vi "VMS View.vi"() -> ()   [LabVIEW 2016, in "M1M3SupportEUI_Views.lvlib"]
uses:
  M1M3SupportEUI_Views.lvlib
  Model/Model.lvclass
  SALLV_vms/DataTypes/M1M3.ctl
  SALLV_vms/DataTypes/logevent_AcquisitionRate.ctl
  SALLV_vms/DataTypes/logevent_AppliedSettingsMatchStart.ctl
  SALLV_vms/DataTypes/logevent_ErrorCode.ctl
  SALLV_vms/DataTypes/logevent_SettingVersions.ctl
  SALLV_vms/DataTypes/logevent_SummaryState.ctl
  M1M3 Support Events/M1M3 Support Events.lvclass/M1M3 Support Events.ctl
  M1M3 Support Events/M1M3 Support Events.lvclass
  SALLV_vms/SALLV_vms.lvlib
panel:
  out "VMS Summary State Value":T1(ring)
  out "Recommended Settings Version":string
  out "Error Code":i32
  out "Applied Settings Match Start":bool
  out "Acquisition Rate":dbl
  out "Acquisition Rate Timestamp":timestamp
  out "Stop":bool
  out "logevent_SummaryState":T2
  out "logevent_SettingVersions":T3
  out "logevent_ErrorCode":T4
  out "logevent_AppliedSettingsMatchStart":T5
  out "logevent_AcquisitionRate":T6
  out "Array":dbl[][](array[numeric])
  in  "Topic":string(combo)
  out "Timestamp":timestamp
  out "M1M3":T7
  in  "Model in":refnum<class "Model.lvclass">
  # "VMS"
  # "Data"
  # "0"
  # "1"
  # "2"
  # "3"
  # "4"
  # "5"
  # "6"
  # "7"
  # "8"
  # "9"
  # "00"
  # "10"
  # "20"
  # "30"
  # "40"
  # "Events"
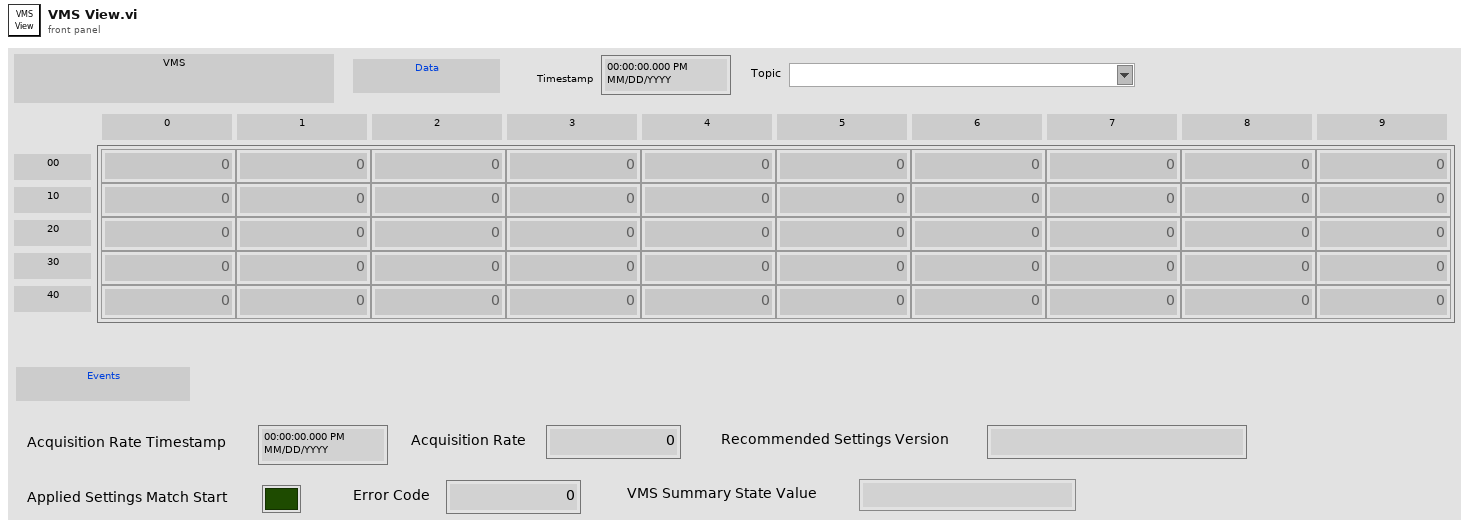
[diagram p1: front panel]
types:
  T1 = enum16{"", "DisabledState", "EnabledState", "FaultState", "OfflineState", "StandbyState"}
  T2 = typedef "SALLV_vms.lvlib/logevent_SummaryState.ctl" = cluster{"SummaryStateValue":enum16{"", "DisabledState", "EnabledState", "FaultState", "OfflineState", "StandbyState"}, "priority":i32}
  T3 = typedef "SALLV_vms.lvlib/logevent_SettingVersions.ctl" = cluster{"recommendedSettingVersion":string, "priority":i32}
  T4 = typedef "SALLV_vms.lvlib/logevent_ErrorCode.ctl" = cluster{"errorCode":i32, "priority":i32}
  T5 = typedef "SALLV_vms.lvlib/logevent_AppliedSettingsMatchStart.ctl" = cluster{"appliedSettingsMatchStartIsTrue":bool, "priority":i32}
  T6 = typedef "SALLV_vms.lvlib/logevent_AcquisitionRate.ctl" = cluster{"Timestamp":dbl, "RateInHz":dbl, "priority":i32}
  T7 = typedef "SALLV_vms.lvlib/M1M3.ctl" = cluster{"Timestamp":dbl, "Sensor1XAcceleration[50]":dbl[], "Sensor1YAcceleration[50]":dbl[], "Sensor1ZAcceleration[50]":dbl[], "Sensor2XAcceleration[50]":dbl[], "Sensor2YAcceleration[50]":dbl[], "Sensor2ZAcceleration[50]":dbl[], "Sensor3XAcceleration[50]":dbl[], "Sensor3YAcceleration[50]":dbl[], "Sensor3ZAcceleration[50]":dbl[]}
  T8 = typedef "M1M3SupportEUI_TypeDefs.lvlib/M1M3 Support Events.ctl" = cluster{"Inclinometer  Data":refnum<user-event>, "IMS Data":refnum<user-event>, "SAL Connected":refnum<user-event>, "Accelerometer Data":refnum<user-event>, "OuterLoop Data":refnum<user-event>, "ErrorCode Event":refnum<user-event>, "InterlockStatus Event":refnum<user-event>, "InterlockWarning Event":refnum<user-event>, "Gyro Data":refnum<user-event>, "HP Actuator Info Event":refnum<user-event>, " FA Info Event":refnum<user-event>, "HP Monitor Info Event":refnum<user-event>, "FA Data":refnum<user-event>, "HP Actuator data":refnum<user-event>, "HP Monitor data":refnum<user-event>, "Air Supply Status Event":refnum<user-event>, "Air Supply Warning Event":refnum<user-event>, "Power Data":refnum<user-event>, "PID Data":refnum<user-event>, "PID Info Event":refnum<user-event>, "Power Status Event":refnum<user-event>, "Power Supply Status Event":refnum<user-event>, "Power Warning Event":refnum<user-event>, "Summary State Event":refnum<user-event>, "Detailed State Event":refnum<user-event>, "FA Force Warning Event":refnum<user-event>, "FA Warning Event":refnum<user-event>, "FA State Event":refnum<user-event>, "Applied AberrationForces Event":refnum<user-event>, "Applied Acceleration Forcces Event":refnum<user-event>, "Applied Azimuth Forces Event":refnum<user-event>, "Applied Active Optic Forces Event":refnum<user-event>, "Applied Balance Forces Event":refnum<user-event>, "Applied Cylinder Forces Event":refnum<user-event>, "Applied Elevation Forces Event":refnum<user-event>, "Applied Forces Event":refnum<user-event>, "Applied Offset Forces Event":refnum<user-event>, "Applied Static Forces Event":refnum<user-event>, "Applied Thermal Forces Event":refnum<user-event>, "Applied Velocity Forces Event":refnum<user-event>, "Rejected Aberration Force Event":refnum<user-event>, "Rejected Acceleration Forces Event":refnum<user-event>, "Rejected Active Optic Forces Event":refnum<user-event>, "Rejected Azimuth Forces Event":refnum<user-event>, "Rejected Balance Forces Event":refnum<user-event>, "Rejected Cylinder Forces Event":refnum<user-event>, "Rejected Elevation Forces Event":refnum<user-event>, "Rejected Forces Event":refnum<user-event>, "Rejected Offset Forces Event":refnum<user-event>, "Rejected Static Forces Event":refnum<user-event>, "Rejected Thermal Forces Event":refnum<user-event>, "Rejected Velocity Forces Event":refnum<user-event>, "Command Rejection Event":refnum<user-event>, "Setting Verions Event":refnum<user-event>, "Settings Applied Event":refnum<user-event>, "HP Actuator State Event":refnum<user-event>, "HP Actuator Warning Event":refnum<user-event>, "HP Monitor State Event":refnum<user-event>, "HP Monitor Warning Event":refnum<user-event>, "Accelerometer Warning Event":refnum<user-event>, "Applied Settings Match Start Event":refnum<user-event>, "Cell Light Status Event ":refnum<user-event>, "Cell Light Warning Event":refnum<user-event>, "Displacement Sensor Warning Event":refnum<user-event>, "Force Setpoint Warning Event":refnum<user-event>, "Gyro Warning Event ":refnum<user-event>, "ILC Warning Event ":refnum<user-event>, "Inclinometer Sensor Warning Event ":refnum<user-event>, "vms M1M3 Data":refnum<user-event>, "vms Acquisition Rate Event":refnum<user-event>, "vms Applied Settings Match Settings Event":refnum<user-event>, "vms Error Code Event":refnum<user-event>, "vms Setting Versions Event":refnum<user-event>, "vms Summary State Event":refnum<user-event>}
  T9 = enum16{"", "DetailedState_DetailedStates_DisabledState", "DetailedState_DetailedStates_EnabledState", "DetailedState_DetailedStates_FaultState", "DetailedState_DetailedStates_OfflineState", "DetailedState_DetailedStates_StandbyState", "DetailedState_DetailedStates_ParkedState", "DetailedState_DetailedStates_RaisingState", "DetailedState_DetailedStates_ActiveState", "DetailedState_DetailedStates_LoweringState", "DetailedState_DetailedStates_EngineeringState", "DetailedState_DetailedStates_ParkedEngineeringState", "DetailedState_DetailedStates_RaisingEngineeringState", "DetailedState_DetailedStates_ActiveEngineeringState", "DetailedState_DetailedStates_LoweringEngineeringState", "DetailedState_DetailedStates_LoweringFaultState", "DetailedState_DetailedStates_ProfileHardpointCorrectionState"}
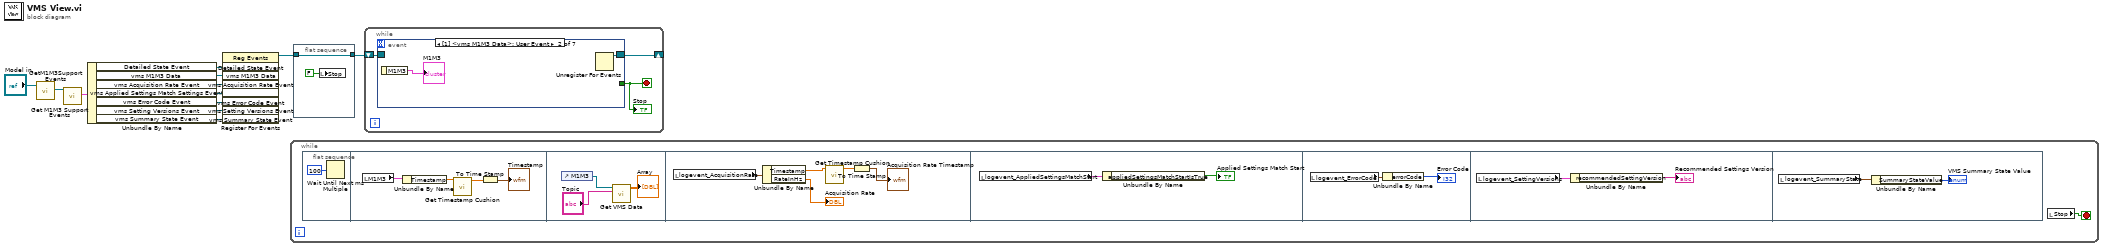
[diagram p0: block diagram]
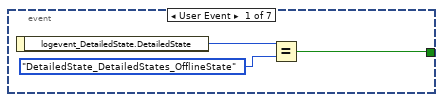
[diagram p2: hidden frame]
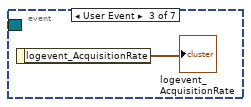
[diagram p3: hidden frame]
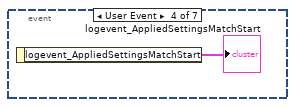
[diagram p4: hidden frame]
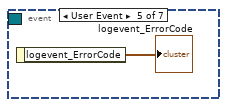
[diagram p5: hidden frame]
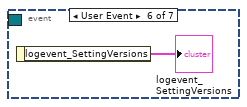
[diagram p6: hidden frame]
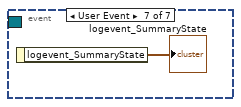
[diagram p7: hidden frame]
diagram:
  n1 = call "GetM1M3SupportEvents.vi"("Model in"="Model in") -> ("M1M3 Support Events out"=w13:refnum<class "M1M3 Support Events.lvclass">)  [unwired: 8 in, 2 out]
  n2 = call "Get M1M3 Support Events.vi"("M1M3 Support Events in"=w13) -> ("M1M3 Support Events"=w11:T8)  [unwired: 9 in, 1 out]
  n3 = Unbundle By Name(w11) -> ("Detailed State Event"=w10:refnum<user-event>, "vms M1M3 Data"=w8:refnum<user-event>, "vms Acquisition Rate Event"=w7:refnum<user-event>, "vms Applied Settings Match Settings Event"=w6:refnum<user-event>, "vms Error Code Event"=w5:refnum<user-event>, "vms Setting Versions Event"=w4:refnum<user-event>, "vms Summary State Event"=w3:refnum<user-event>)
  n4 = register-events(w10, w8, w7, w6, w5, w4, w3) -> (reference out=w2:refnum<event-registration>)  [unwired: 2 in, 1 out]
  n5 = while {
    stop <- w14 stop-if-true
    n6 = flat-sequence {
      frame #0 {
        n7 = Wait Until Next ms Multiple(millisecond multiple=u32 100) -> ()  [unwired: 1 out]
      }
      frame #1 {
        n8 = local read "M1M3"() -> (w19:T7)
        n9 = Unbundle By Name(w19) -> ("Timestamp"=w17:dbl)
        n10 = call "Get Timestamp Cushion.vi"("DoubleTimestampRepresentation"=w17) -> ("TimestampCushion"=w18:dbl)  [unwired: 10 in]
        n11 = To Time Stamp(1:w18) -> (0:→"Timestamp":timestamp)
      }
      frame #2 {
        n12 = control-ref of="M1M3"() -> (w22:refnum<vi>)
        n13 = call "Get VMS Data.vi"("VMS Data Type"="Topic", "Clust Refnum"=w22) -> ("Array"=→"Array":dbl[][])  [unwired: 9 in]
      }
      frame #3 {
        n14 = local read "logevent_AcquisitionRate"() -> (w27:T6)
        n15 = Unbundle By Name(w27) -> ("Timestamp"=w25:dbl, "RateInHz"=→"Acquisition Rate":dbl)
        n16 = call "Get Timestamp Cushion.vi"("DoubleTimestampRepresentation"=w25) -> ("TimestampCushion"=w26:dbl)  [unwired: 10 in]
        n17 = To Time Stamp(1:w26) -> (0:→"Acquisition Rate Timestamp":timestamp)
      }
      frame #4 {
        n18 = local read "logevent_AppliedSettingsMatchStart"() -> (w29:T5)
        n19 = Unbundle By Name(w29) -> ("appliedSettingsMatchStartIsTrue"=→"Applied Settings Match Start":bool)
      }
      frame #5 {
        n20 = local read "logevent_ErrorCode"() -> (w31:T4)
        n21 = Unbundle By Name(w31) -> ("errorCode"=→"Error Code":i32)
      }
      frame #6 {
        n22 = local read "logevent_SettingVersions"() -> (w33:T3)
        n23 = Unbundle By Name(w33) -> ("recommendedSettingVersion"=→"Recommended Settings Version":string)
      }
      frame #7 {
        n24 = local read "logevent_SummaryState"() -> (w35:T2)
        n25 = Unbundle By Name(w35) -> ("SummaryStateValue"=→"VMS Summary State Value":T1)
      }
    }
    n26 = local read "Stop"() -> (w14:bool)
  }
  n27 = flat-sequence {
    tunnel: w2 -> [w37]
    tunnel: [w37] -> w1
    frame #0 {
      n28 = local write "Stop"(FALSE ("Stop")) -> ()
    }
  }
  n29 = while {
    shift-right: [w39] -> w9
    shift-left: w1 -> [w40]
    stop <- w38 stop-if-true
    n30 = event shown="[1] <vms M1M3 Data>: User Event" {
      selector: w40 -> [_ _ _ _ _ _ _]
      dyn-events: [_ _ _ _ _ _ _] -> w39
      timeout: _ -> [_ _ _ _ _ _ _]
      tunnel: [w41 _ _ _ _ _ _] -> w38
      event User Event {
        n31 = event-data() -> ("logevent_DetailedState.DetailedState"=w43:T9)  [unwired: 1 in]
        n32 = Equal?(x=w43, y=T9."DetailedState_DetailedStates_OfflineState") -> (x = y?=w41:bool)
      }
      event User Event {
        n33 = event-data() -> ("M1M3"=→"M1M3":T7)  [unwired: 1 in]
      }
      event User Event {
        n34 = event-data() -> ("logevent_AcquisitionRate"=→"logevent_AcquisitionRate":T6)  [unwired: 1 in]
      }
      event User Event {
        n35 = event-data() -> ("logevent_AppliedSettingsMatchStart"=→"logevent_AppliedSettingsMatchStart":T5)  [unwired: 1 in]
      }
      event User Event {
        n36 = event-data() -> ("logevent_ErrorCode"=→"logevent_ErrorCode":T4)  [unwired: 1 in]
      }
      event User Event {
        n37 = event-data() -> ("logevent_SettingVersions"=→"logevent_SettingVersions":T3)  [unwired: 1 in]
      }
      event User Event {
        n38 = event-data() -> ("logevent_SummaryState"=→"logevent_SummaryState":T2)  [unwired: 1 in]
      }
    }
    "Stop" <- w38
  }
  n39 = Unregister For Events(event registration refnum=w9) -> ()  [unwired: 1 in, 1 out]
